vi "rtp play.vi"(4 "voltage range":dbl, 6 "freq":u32, 7 "rtp stop event ref":refnum<user-event>, 8 "error in (no error)":errorcluster caption="에러 입력(에러 없음)", 10 "waveform data":i8[](array[numeric]), 11 "DW7800 입력":refnum<class "DW7800.lvclass">) -> (0 "error out":errorcluster caption="에러 출력", 3 "DW7800 출력":refnum<class "DW7800.lvclass">)   [LabVIEW 2020, in "DW7800.lvclass"]
uses:
  DW7800.lvclass
  Haptic IC/Haptic IC.lvclass/Haptic IC.ctl
  SubVIs/I2C/Instance VIs/(SubVI)I2C_8Bit-8Bit_Read_Single.vi
  SubVIs/I2C/Instance VIs/(SubVI)I2C_8Bit-8Bit_Write_Single.vi
  Haptic IC/Haptic IC.lvclass
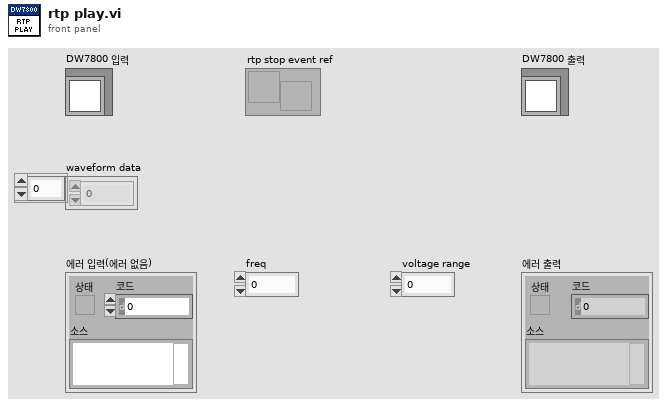
[diagram p1: front panel]
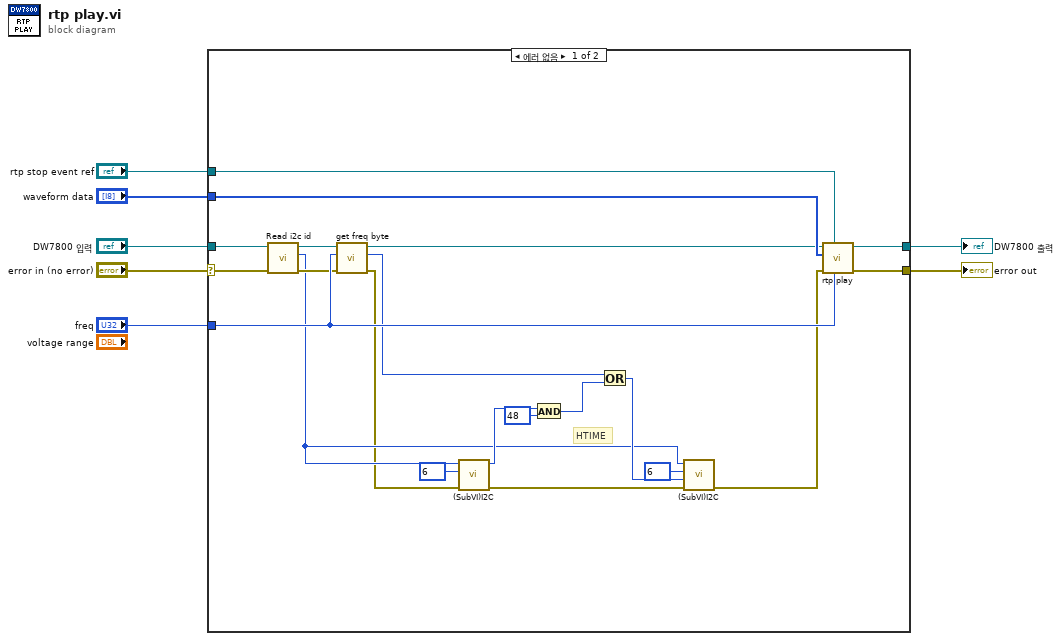
[diagram p0: block diagram]
diagram:
  n1 = case shown="에러 없음" "error in (no error)" {
    selector: "error in (no error)" -> [w25 w29]
    tunnel: [w28 w29] -> w7
    tunnel: [w27 w30] -> w6
    tunnel: "freq" -> [w22 _]
    tunnel: "rtp stop event ref" -> [w26 _]
    tunnel: "waveform data" -> [w24 _]
    tunnel: "DW7800 입력" -> [w20 w30]
    frame No Error {
      # "HTIME"
      n2 = call "Read i2c id.vi"("error in (no error)"=w25, "Haptic IC 입력"=w20) -> ("error out"=w21:errorcluster, "i2c id"=w11:u8, "Haptic IC 출력"=w19:refnum<class "DW7800.lvclass">)  [unwired: 7 in]
      n3 = call-dynamic "get freq byte.vi"("error in (no error)"=w21, "freq"=w22, "DW7800 입력"=w19) -> ("error out"=w10:errorcluster, "byte value"=w8:u8, "DW7800 출력"=w23:refnum<class "DW7800.lvclass">)  [unwired: 6 in]
      n4 = call-poly "(SubVI)I2C.vi"("error in (no error)"=w10, "Address"=u8 6, "ID"=w11) -> ("error out"=w13:errorcluster, "Read Data"=w17:u8)  [unwired: 6 in, 1 out]
      n5 = And(x=w17, y=u8 48) -> (x .and. y?=w15:u8)
      n6 = Or(x=w8, y=w15) -> (x .or. y?=w12:u8)
      n7 = call-poly "(SubVI)I2C.vi"("error in (no error)"=w13, "Data to Write"=w12, "Address"=u8 6, "ID"=w11) -> ("error out"=w9:errorcluster)  [unwired: 6 in, 1 out]
      n8 = call-parent "rtp play.vi"("freq"=w22, "rtp stop event ref"=w26, "error in (no error)"=w9, "waveform data"=w24, "Haptic IC 입력"=w23) -> ("error out"=w28:errorcluster, "Haptic IC 출력"=w27:refnum<class "DW7800.lvclass">)  [unwired: 5 in]
    }
    frame Error {
    }
  }
  "error out" <- w7
  "DW7800 출력" <- w6
